vi "RP100MeasVolt.vi"(3 "error in (no error)":errorcluster, 4 "Source":enum16{"1", "2"}(ring), 5 "VISA resource name":refnum<visa-resource-name>) -> (0 "error out":errorcluster, 1 "Voltage":dbl, 2 "VISA resource name out":refnum<visa-resource-name>)   [LabVIEW 2023]
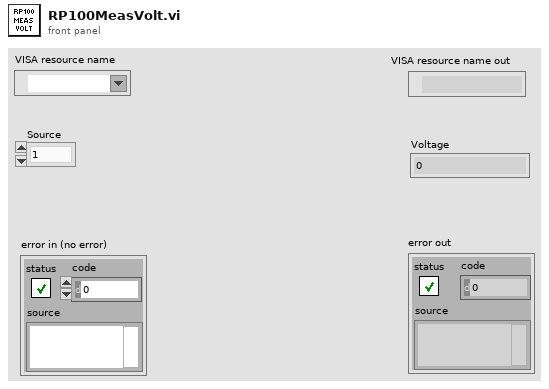
[diagram p1: front panel]
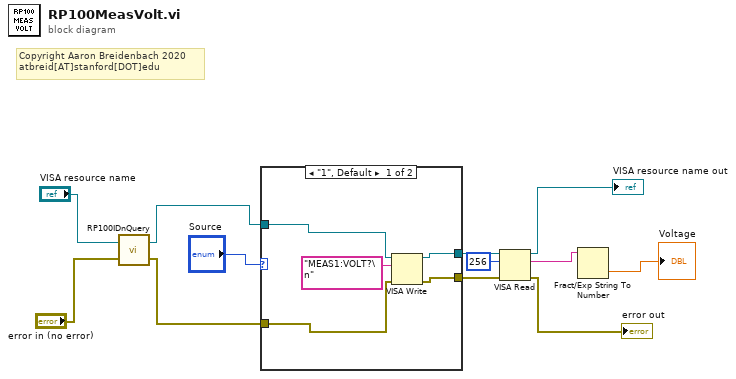
[diagram p0: block diagram]
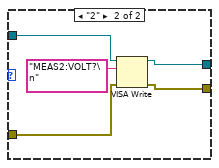
[diagram p2: hidden frame]
diagram:
  # "Copyright Aaron Breidenbach 2020\natbreid[AT]stanford[DOT]edu"
  n1 = call "RP100IDnQuery.vi"("error in (no error)"="error in (no error)", "VISA resource name"="VISA resource name") -> ("error out"=w1:errorcluster, "VISA resource name out"=w2:refnum<visa-resource-name>)
  n2 = case shown="\"1\", Default" "Source" {
    tunnel: w2 -> [w16 w22]
    tunnel: w1 -> [w15 w21]
    tunnel: [w14 w19] -> w11
    tunnel: [w13 w18] -> w10
    frame "1", Default {
      n3 = VISA Write(VISA resource name=w16, write buffer="MEAS1:VOLT?\n", error in (no error)=w15) -> (VISA resource name out=w14:refnum<visa-resource-name>, error out=w13:errorcluster)  [unwired: 1 out]
    }
    frame "2" {
      n4 = VISA Write(VISA resource name=w22, write buffer="MEAS2:VOLT?\n", error in (no error)=w21) -> (VISA resource name out=w19:refnum<visa-resource-name>, error out=w18:errorcluster)  [unwired: 1 out]
    }
  }
  n5 = VISA Read(VISA resource name=w11, byte count=u32 256, error in (no error)=w10) -> (VISA resource name out=→"VISA resource name out":refnum<visa-resource-name>, read buffer=w6:string, error out=→"error out":errorcluster)  [unwired: 1 out]
  n6 = Fract/Exp String To Number(string=w6) -> (number=→"Voltage":dbl)  [unwired: 3 in, 1 out]
